vi "Stato comandi freno.vi"() -> ()   [LabVIEW 2019]
uses:
  TypeDef/Stato inverter selezionato.ctl
  TypeDef/Comandi freno.ctl
panel:
  out "RPM max freno":dbl
  out "Cmax freno":dbl
  out "Stato inverter":T1
  # "CHANGING CONTROL\nTYPE...."
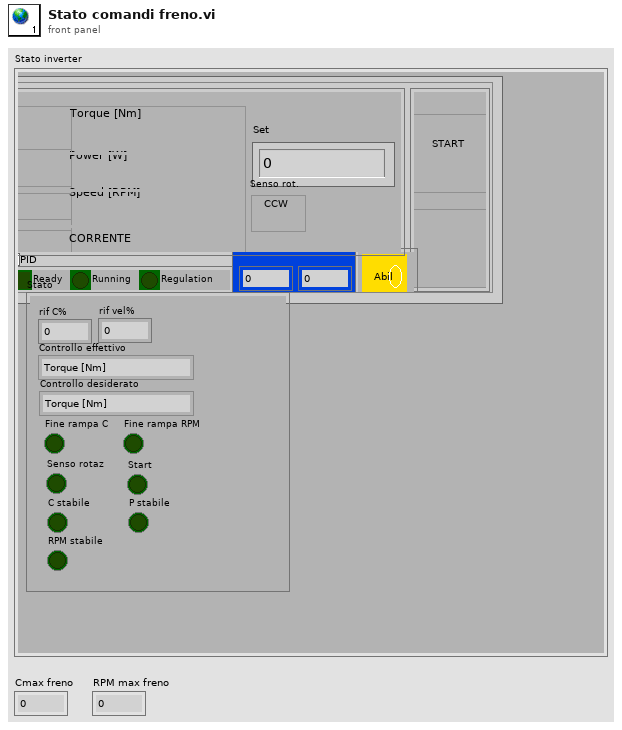
[diagram p1: front panel]
types:
  T1 = typedef "Stato inverter selezionato.ctl" = cluster{"Stato comandi freno":T2, "Stato":cluster{"rif C%":dbl, "rif vel%":dbl, "Controllo effettivo":enum32{"Torque [Nm]", "Power [W]", "Speed [RPM]"}, "Controllo desiderato":enum32{"Torque [Nm]", "Power [W]", "Speed [RPM]"}, "Fine rampa C":bool, "Fine rampa RPM":bool, "Senso rotaz":bool, "Start":bool, "C stabile":bool, "P stabile":bool, "RPM stabile":bool}}
  T2 = typedef "Comandi freno.ctl" = cluster{"Control":cluster{"Control Type":enum32{"Torque [Nm]", "Power [W]", "Speed [RPM]", "Corrente [A]"}, "Set":dbl, "Inverti senso di rotazione":bool}, "Start\\stop":cluster{"Start":bool, "STOP":bool}, "Status":cluster{"Ready":bool, "Running":bool, "Regulation":bool}, "PID":bool, "Abilita":cluster{"Abilita":bool}, "Status ref":cluster{"Torque":dbl, "Speed":dbl}}
diagram:
